vi "PhotonUtils_EstimateCameraToTarget.vi"(9 "GyroAngle":T3={"VALUE"=0.0, "COS"=1.0, "SIN"=0.0} {"SIN" format="%13.4f"; "COS" format="%13.4f"; "VALUE" format="%13.4f"}, 10 "FieldToTarget":T4={"TRANSLATION"={"X"=0.0, "Y"=0.0}, "ROTATION"={"VALUE"=0.0, "COS"=1.0, "SIN"=0.0}} {"ROTATION"."SIN" format="%13.4f"; "ROTATION"."COS" format="%13.4f"; "ROTATION"."VALUE" format="%13.4f"; "TRANSLATION"."Y" format="%14.3f"; "TRANSLATION"."X" format="%14.3f"}, 11 "CameraToTargetTranslation":T2 {"Y" format="%14.3f"; "X" format="%14.3f"}) -> (3 "estimateCameraToTarget":T1 {"ROTATION"."SIN" format="%13.4f"; "ROTATION"."COS" format="%13.4f"; "ROTATION"."VALUE" format="%13.4f"; "TRANSLATION"."Y" format="%14.3f"; "TRANSLATION"."X" format="%14.3f"})   [LabVIEW 2020, in "PhotonVisionLib.lvlib"]
doc: "Estimates a Transform2d that maps the camera position to the target position, using the robot's gyro. Note that the gyro angle provided *must* line up with the field coordinate system -- that is, it should read zero degrees when pointed towards the opposing alliance station, and increase as the robot rotates CCW.\n \nInputs: \n - CameraToTargetTranslation -- A Translation2d that encodes the x/y position \n of the target relative to the camera.\n - FieldToTarget -- A Pose2d representing the target position in the field coordinate \n system.\n - GyroAngle -- The current robot gyro angle, likely from odometry.\n\nOutputs:\n - EstimateCameraToTarget -- A Transform2d that takes us from the camera to \n the target."
uses:
  PhotonVisionLib.lvlib
  <vilib>/Rock Robotics/WPI/ThirdParty/JAS_Junk/TrajLib/TypeDef/TRANSLATION2D.ctl
  <vilib>/Rock Robotics/WPI/ThirdParty/JAS_Junk/TrajLib/TypeDef/POSE2D.ctl
  <vilib>/Rock Robotics/WPI/ThirdParty/JAS_Junk/TrajLib/TypeDef/ROTATION2D.ctl
  <vilib>/Rock Robotics/WPI/ThirdParty/JAS_Junk/TrajLib/TypeDef/TRANSFORM2D.ctl
  <vilib>/Rock Robotics/WPI/ThirdParty/JAS_Junk/TrajLib/Rotation2d_CreateAngle.vi
  <vilib>/Rock Robotics/WPI/ThirdParty/JAS_Junk/TrajLib/Rotation2d_UnaryMinus.vi
  <vilib>/Rock Robotics/WPI/ThirdParty/JAS_Junk/TrajLib/Rotation2d_RotateBy.vi
  <vilib>/Rock Robotics/WPI/ThirdParty/JAS_Junk/TrajLib/Rotation2d_CreateXY.vi
  <vilib>/Rock Robotics/WPI/ThirdParty/JAS_Junk/TrajLib/Util_CalcDist.vi
  <vilib>/Rock Robotics/WPI/ThirdParty/JAS_Junk/TrajLib/Trajectory_Library.lvlib
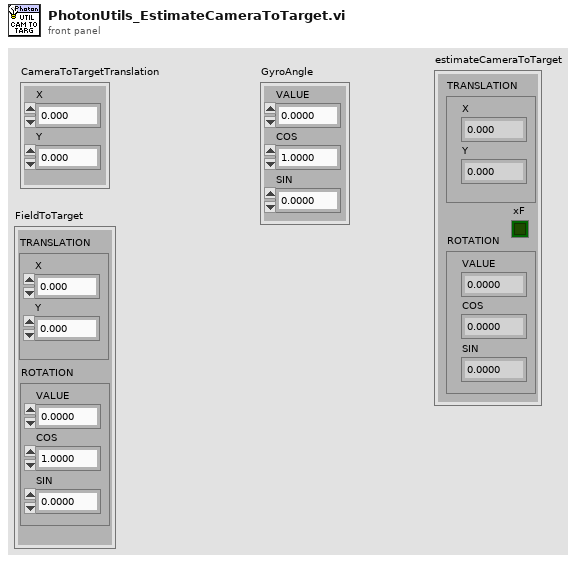
[diagram p1: front panel]
types:
  T1 = typedef "Trajectory_Library.lvlib/TRANSFORM2D.ctl" = cluster{"TRANSLATION":T2, "ROTATION":T3, "xF":bool}
  T2 = typedef "Trajectory_Library.lvlib/TRANSLATION2D.ctl" = cluster{"X":dbl, "Y":dbl}
  T3 = typedef "Trajectory_Library.lvlib/ROTATION2D.ctl" = cluster{"VALUE":dbl, "COS":dbl, "SIN":dbl}
  T4 = typedef "Trajectory_Library.lvlib/POSE2D.ctl" = cluster{"TRANSLATION":T2, "ROTATION":T3}
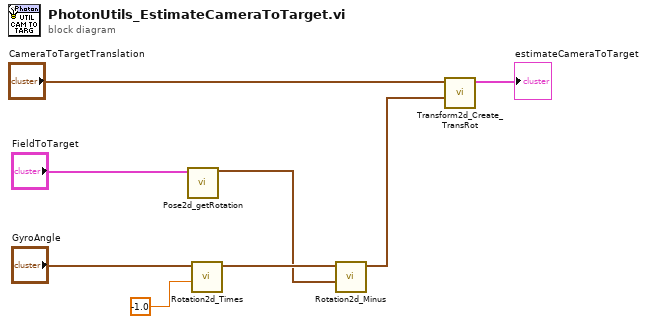
[diagram p0: block diagram]
diagram:
  n1 = call <vilib>:"Pose2d_getRotation.vi"("in POSE"="FieldToTarget") -> ("out ROTATION"=w4:T3)  [unwired: 10 in]
  n2 = call <vilib>:"Rotation2d_Times.vi"("Scalar"=-1.0, "in ROTATION"="GyroAngle") -> ("out ROTATION"=w5:T3)  [unwired: 9 in]
  n3 = call <vilib>:"Rotation2d_Minus.vi"("other ROTATION"=w4, "in ROTATION"=w5) -> ("out ROTATION"=w2:T3)  [unwired: 9 in]
  n4 = call <vilib>:"Transform2d_Create_TransRot.vi"("ROTATION"=w2, "TRANSLATION"="CameraToTargetTranslation") -> ("TRANSFORM"=→"estimateCameraToTarget":T1)  [unwired: 9 in]
